vi "Main.vi"() -> ()   [LabVIEW 2020]
uses:
  <vilib>/High Genius/HG_WSI_Tookit/Dependencies/Library/CAN/CAN.lvclass
  C:/Program Files (x86)/National Instruments/LabVIEW 2020/vi.lib/High Genius/HG_WSI_Tookit/Dependencies/Library/HG_LIB/HG_LIB.lvclass
  <vilib>/High Genius/HG_WSI_Tookit/Dependencies/Library/PWM/PWM.lvclass
  <vilib>/High Genius/HG_WSI_Tookit/Dependencies/Library/Analog In/Analog In.lvclass
  <vilib>/High Genius/HG_WSI_Tookit/Dependencies/Library/Pulse/Pulse.lvclass
  <vilib>/High Genius/HG_WSI_Tookit/Dependencies/Library/ISQ/ISQ.lvclass
  <vilib>/High Genius/HG_WSI_Tookit/Dependencies/Library/IIC/IIC.lvclass
  <vilib>/High Genius/HG_WSI_Tookit/Dependencies/Library/IMU/IMU.lvclass
  <vilib>/High Genius/HG_WSI_Tookit/Dependencies/Library/Digital Input and Output/Digital Input and Output.lvclass
  <vilib>/Platform/TimedLoop/XDataNode/timing_clust.ctl
  <vilib>/Platform/TimedLoop/XDataNode/nitl_modes.ctl
  <vilib>/Platform/TimedLoop/XDataNode/wakeup.ctl
  <vilib>/Platform/TimedLoop/XDataNode/XDataNode.xnode
  <vilib>/High Genius/HG_WSI_Tookit/Dependencies/Library/HG_LIB/HG_LIB.lvclass
  <vilib>/Platform/TimedLoop/XDataNode/XDNodeRunTimeDep.lvlib
panel:
  in  "Reset Yaw":bool
  out "NavX Yaw (Rad)":dbl
  out "Ultrasonic Distance":dbl
  out "Sharp IR Distance":dbl
  out "Sharp IR Voltage":dbl
  in  "Stop Button":bool
  in  "In A":bool
  in  "In B":bool
  in  "Motor Duty Cycle":dbl(slide) scale=0.0..255.0
  out "NavX Data":dbl[](array[numeric])
  out "Cobra Values":dbl[](array[numeric])
  out "Push Button":bool
  out "Loop Number":i32
  in  "Ultrasonic Pulse":i32=20 min=0 step=1
  in  "Servo PWM":dbl(slide) min=-150.0 max=255.0 step=1.0 scale=-150.0..150.0
  # "S1"
  # "S2"
  # "S3"
  # "S4"
  # "Yaw"
  # "Pitch"
  # "Roll"
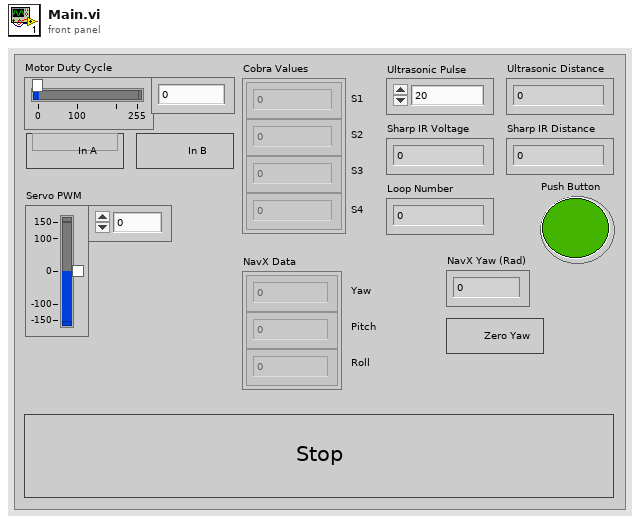
[diagram p1: front panel]
types:
  T1 = enum16{"0", "1", "2", "3", "4", "5", "6", "7", "8", "9", "10", "11", "12", "13", "14", "15", "16", "17", "18", "19", "20", "21", "22", "23", "24", "25"}
  T2 = enum16{"DI", "DO", "AI", "Pulse", "PWM", "ISQ", "ENC", "CAN", "IIC", "IMU"}
  T3 = typedef "XDNodeRunTimeDep.lvlib/timing_clust.ctl" = cluster{"Expected End [f-1]":u64, "Actual End [f-1]":u64, "Finished Late? [f-1]":bool, "Expected End [i-1]":u64, "Actual End [i-1]":u64, "Finished Late? [i-1]":bool, "Expected Start [i]":u64, "Actual Start [i]":u64, "Expected Start [f]":u64, "Actual Start [f]":u64, "Source Name":string, "Structure Name":string, "Period":i64, "Deadline":i64, "Offset":i64, "Start":i64, "Priority":i32, "Timeout":i32, "Mode":T4, "Wakeup Reason":T5, "Error":errorcluster, "Source Type":string, "Secondary Source Type":string, "Global End Time":u64, "Global Start Time":u64, "Frame Duration":u64, "Iteration Duration":u64, "Assigned CPU":i32, "I/O Scan Engine Mode":u32}
  T4 = typedef "XDNodeRunTimeDep.lvlib/nitl_modes.ctl" = enum32{"No Change", "Process missed periods, maintain original phase", "Discard missed periods, maintain original phase", "Process missed periods, ignore original phase", "Discard missed periods, ignore original phase"}
  T5 = typedef "XDNodeRunTimeDep.lvlib/wakeup.ctl" = enum32{"Normal", "Aborted", "Asynchronous wakeup", "Timing source error", "Timed loop error", "Timeout"}
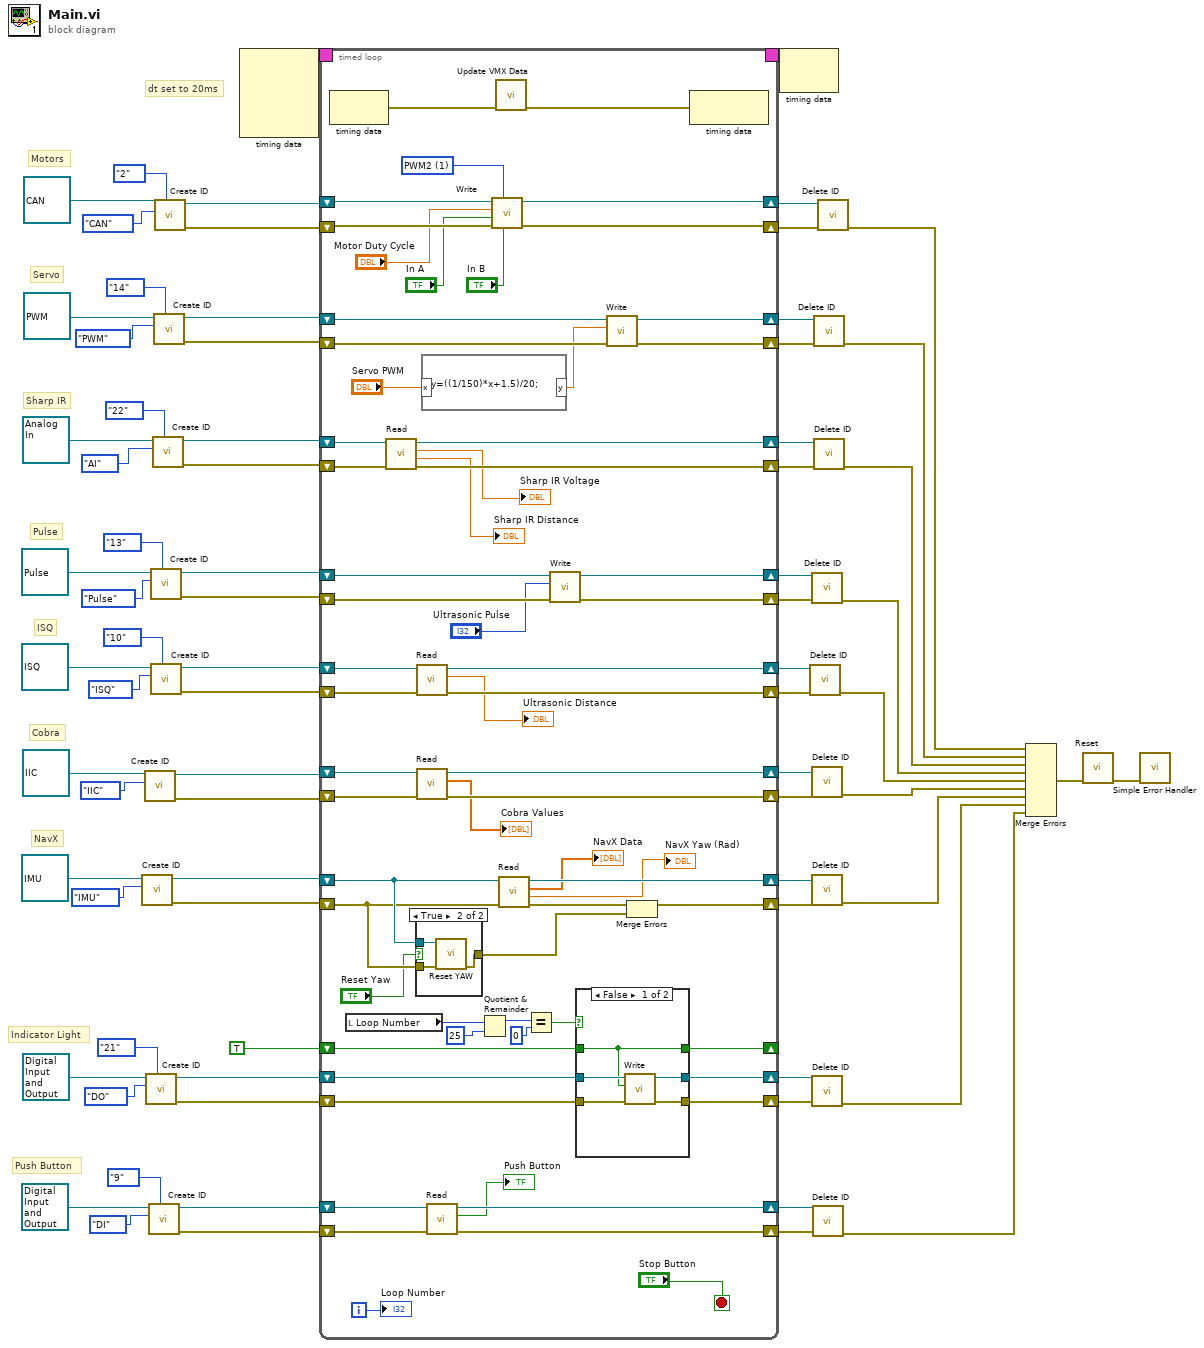
[diagram p0: block diagram]
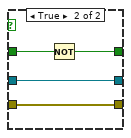
[diagram p2: hidden frame]
diagram:
  # "Push Button"
  # "Indicator Light"
  # "NavX"
  # "Cobra"
  # "ISQ"
  # "Pulse"
  # "Sharp IR"
  # "Servo"
  # "Motors"
  # "dt set to 20ms"
  n1 = call <vilib>:"Create ID.vi"("Function"=T2."IMU", "HG_LIB in"=refnum<class "IMU.lvclass"> refnum ("VMX Library.lvlib:IMU.lvclass")) -> ("error out"=w19:errorcluster, "HG_LIB out"=w20:refnum<class "IMU.lvclass">)  [unwired: 8 in]
  n2 = call <vilib>:"Create ID.vi"("Function"=T2."IIC", "HG_LIB in"=refnum<class "IIC.lvclass"> refnum ("VMX Library.lvlib:IIC.lvclass")) -> ("error out"=w26:errorcluster, "HG_LIB out"=w27:refnum<class "IIC.lvclass">)  [unwired: 8 in]
  n3 = call <vilib>:"Create ID.vi"("NO"=T1."21", "Function"=T2."DO", "HG_LIB in"=refnum<class "Digital Input and Output.lvclass"> refnum ("VMX Library.lvlib:Digital Input and Output.lvclass")) -> ("error out"=w10:errorcluster, "HG_LIB out"=w11:refnum<class "Digital Input and Output.lvclass">)  [unwired: 7 in]
  n4 = call <vilib>:"Create ID.vi"("NO"=T1."9", "Function"=T2."DI", "HG_LIB in"=refnum<class "Digital Input and Output.lvclass"> refnum ("VMX Library.lvlib:Digital Input and Output.lvclass")) -> ("error out"=w2:errorcluster, "HG_LIB out"=w3:refnum<class "Digital Input and Output.lvclass">)  [unwired: 7 in]
  n5 = call <vilib>:"Create ID.vi"("NO"=T1."13", "Function"=T2."Pulse", "HG_LIB in"=refnum<class "Pulse.lvclass"> refnum ("VMX Library.lvlib:Pulse.lvclass")) -> ("error out"=w42:errorcluster, "HG_LIB out"=w43:refnum<class "Pulse.lvclass">)  [unwired: 7 in]
  n6 = call <vilib>:"Create ID.vi"("NO"=T1."10", "Function"=T2."ISQ", "HG_LIB in"=refnum<class "ISQ.lvclass"> refnum ("VMX Library.lvlib:ISQ.lvclass")) -> ("error out"=w36:errorcluster, "HG_LIB out"=w37:refnum<class "ISQ.lvclass">)  [unwired: 7 in]
  n7 = call <vilib>:"Create ID.vi"("NO"=T1."22", "Function"=T2."AI", "HG_LIB in"=refnum<class "Analog In.lvclass"> refnum ("VMX Library.lvlib:Analog In.lvclass")) -> ("error out"=w49:errorcluster, "HG_LIB out"=w51:refnum<class "Analog In.lvclass">)  [unwired: 7 in]
  n8 = call <vilib>:"Create ID.vi"("NO"=T1."14", "Function"=T2."PWM", "HG_LIB in"=refnum<class "PWM.lvclass"> refnum ("VMX Library.lvlib:PWM.lvclass")) -> ("error out"=w60:errorcluster, "HG_LIB out"=w59:refnum<class "PWM.lvclass">)  [unwired: 7 in]
  n9 = call <vilib>:"Create ID.vi"("NO"=T1."2", "Function"=T2."CAN", "HG_LIB in"=refnum<class "CAN.lvclass"> refnum ("VMX Library.lvlib:CAN.lvclass")) -> ("error out"=w69:errorcluster, "HG_LIB out"=w68:refnum<class "CAN.lvclass">)  [unwired: 7 in]
  n10 = node-c288() -> (w75:T3)  [unwired: 4 in]
  n11 = timed-loop {
    timing: w75 -> [_]
    timing-out: [_] -> w74
    shift-right: [w136] -> w71
    shift-left: w69 -> [w134]
    shift-right: [w137] -> w72
    shift-left: w68 -> [w135]
    shift-right: [w132] -> w62
    shift-left: w60 -> [w129]
    shift-right: [w131] -> w61
    shift-left: w59 -> [w130]
    shift-right: [w128] -> w52
    shift-left: w51 -> [w127]
    shift-right: [w126] -> w50
    shift-left: w49 -> [w125]
    shift-right: [w124] -> w45
    shift-left: w43 -> [w122]
    shift-right: [w123] -> w44
    shift-left: w42 -> [w121]
    shift-right: [w119] -> w39
    shift-left: w37 -> [w117]
    shift-right: [w118] -> w38
    shift-left: w36 -> [w116]
    shift-right: [w115] -> w29
    shift-left: w27 -> [w113]
    shift-right: [w114] -> w28
    shift-left: w26 -> [w112]
    shift-right: [w111] -> w24
    shift-left: w20 -> [w110]
    shift-right: [w106] -> w23
    shift-left: w19 -> [w109]
    shift-right: [w99] -> _
    shift-left: TRUE -> [w100]
    shift-right: [w98] -> w13
    shift-left: w11 -> [w96]
    shift-right: [w97] -> w12
    shift-left: w10 -> [w95]
    shift-right: [w94] -> w5
    shift-left: w3 -> [w92]
    shift-right: [w93] -> w4
    shift-left: w2 -> [w91]
    i -> [w90]
    stop <- "Stop Button" stop-if-true
    w133 = u16 1 items=["PWM1", "PWM2", "PWM3", "PWM4"] ("PWM")
    n12 = node-c288() -> (w138:errorcluster)  [unwired: 1 in]
    n13 = local read "Loop Number"() -> (w105:i32)
    n14 = call <vilib>:"Read.vi"("error in (no error)"=w125, "Analog In in"=w127) -> ("error out"=w126:errorcluster, "IR"=→"Sharp IR Distance":dbl, "Data"=→"Sharp IR Voltage":dbl, "Analog In out"=w128:refnum<class "Analog In.lvclass">)  [unwired: 6 in]
    n15 = case shown="True" "Reset Yaw" {
      tunnel: w110 -> [_ w152]
      tunnel: w109 -> [w149 w151]
      tunnel: [w149 w150] -> w108
      frame False {
      }
      frame True {
        n16 = call <vilib>:"Reset YAW.vi"("error in (no error)"=w151, "IMU in"=w152) -> ("error out"=w150:errorcluster)  [unwired: 8 in, 1 out]
      }
    }
    n17 = call <vilib>:"Read.vi"("error in (no error)"=w116, "ISQ in"=w117) -> ("error out"=w118:errorcluster, "PING"=→"Ultrasonic Distance":dbl, "ISQ out"=w119:refnum<class "ISQ.lvclass">)  [unwired: 7 in]
    n18 = call <vilib>:"Read.vi"("error in (no error)"=w112, "IIC in"=w113) -> ("error out"=w114:errorcluster, "QTI"=→"Cobra Values":dbl[], "IIC out"=w115:refnum<class "IIC.lvclass">)  [unwired: 7 in]
    n19 = formula code="y=((1/150)*x+1.5)/20;"("x"="Servo PWM") -> ("y"=w76:dbl)
    n20 = call <vilib>:"Read.vi"("error in (no error)"=w91, "Digital Input and Output in"=w92) -> ("error out"=w93:errorcluster, "Boolean"=→"Push Button":bool, "Digital Input and Output out"=w94:refnum<class "Digital Input and Output.lvclass">)  [unwired: 7 in]
    n21 = Quotient & Remainder(x=w105, y=25) -> (x-y*floor(x/y)=w103:i32)  [unwired: 1 out]
    n22 = call <vilib>:"Write.vi"("INB"="In B", "PWM"=w133, "error in (no error)"=w134, "INA"="In A", "Duty Cycle"="Motor Duty Cycle", "CAN in"=w135) -> ("error out"=w136:errorcluster, "CAN out"=w137:refnum<class "CAN.lvclass">)  [unwired: 4 in]
    n23 = call <vilib>:"Update VMX Data.vi"("error in (no error)"=w138) -> ("error out"=w139:errorcluster)  [unwired: 10 in]
    n24 = call <vilib>:"Read.vi"("error in (no error)"=w109, "IMU in"=w110) -> ("error out"=w107:errorcluster, "YAW (rad)"=→"NavX Yaw (Rad)":dbl, "IMU"=→"NavX Data":dbl[], "IMU out"=w111:refnum<class "IMU.lvclass">)  [unwired: 6 in]
    n25 = Equal?(x=w103, y=0) -> (x = y?=w101:bool)
    n26 = call <vilib>:"Write.vi"("error in (no error)"=w121, "Pulse"="Ultrasonic Pulse", "Pulse in"=w122) -> ("error out"=w123:errorcluster, "Pulse out"=w124:refnum<class "Pulse.lvclass">)  [unwired: 7 in]
    n27 = case shown="False" w101 {
      tunnel: w100 -> [w140 w148]
      tunnel: [w140 w147] -> w99
      tunnel: [w144 w146] -> w98
      tunnel: [w143 w145] -> w97
      tunnel: w96 -> [w142 w146]
      tunnel: w95 -> [w141 w145]
      frame False {
        n28 = call <vilib>:"Write.vi"("error in (no error)"=w141, "Control"=w140, "Digital Input and Output in"=w142) -> ("error out"=w143:errorcluster, "Digital Input and Output out"=w144:refnum<class "Digital Input and Output.lvclass">)  [unwired: 7 in]
      }
      frame True {
        n29 = Not(x=w148) -> (.not. x?=w147:bool)
      }
    }
    n30 = call <vilib>:"Write.vi"("error in (no error)"=w129, "PWM"=w76, "PWM in"=w130) -> ("error out"=w132:errorcluster, "PWM out"=w131:refnum<class "PWM.lvclass">)  [unwired: 7 in]
    n31 = Merge Errors(w107, w108) -> (w106:errorcluster)
    n32 = node-c288(w139) -> ()  [unwired: 1 out]
    "Loop Number" <- w90
  }
  n33 = node-c288(w74) -> ()  [unwired: 1 out]
  n34 = call <vilib>:"Delete ID.vi"("error in (no error)"=w38, "HG_LIB in"=w39) -> ("error out"=w32:errorcluster)  [unwired: 8 in, 1 out]
  n35 = call <vilib>:"Delete ID.vi"("error in (no error)"=w44, "HG_LIB in"=w45) -> ("error out"=w33:errorcluster)  [unwired: 8 in, 1 out]
  n36 = call <vilib>:"Delete ID.vi"("error in (no error)"=w28, "HG_LIB in"=w29) -> ("error out"=w25:errorcluster)  [unwired: 8 in, 1 out]
  n37 = call <vilib>:"Delete ID.vi"("error in (no error)"=w23, "HG_LIB in"=w24) -> ("error out"=w18:errorcluster)  [unwired: 8 in, 1 out]
  n38 = call <vilib>:"Delete ID.vi"("error in (no error)"=w12, "HG_LIB in"=w13) -> ("error out"=w9:errorcluster)  [unwired: 8 in, 1 out]
  n39 = call <vilib>:"Delete ID.vi"("error in (no error)"=w4, "HG_LIB in"=w5) -> ("error out"=w1:errorcluster)  [unwired: 8 in, 1 out]
  n40 = call <vilib>:"Delete ID.vi"("error in (no error)"=w62, "HG_LIB in"=w61) -> ("error out"=w63:errorcluster)  [unwired: 8 in, 1 out]
  n41 = call <vilib>:"Delete ID.vi"("error in (no error)"=w50, "HG_LIB in"=w52) -> ("error out"=w48:errorcluster)  [unwired: 8 in, 1 out]
  n42 = call <vilib>:"Delete ID.vi"("error in (no error)"=w71, "HG_LIB in"=w72) -> ("error out"=w64:errorcluster)  [unwired: 8 in, 1 out]
  n43 = Merge Errors(w64, w63, w48, w33, w32, w25, w18, w9, w1) -> (w65:errorcluster)
  n44 = call <vilib>:"Reset.vi"("error in (no error)"=w65) -> ("error out"=w73:errorcluster)  [unwired: 10 in]
  n45 = call <vilib>:"Simple Error Handler.vi"("error in (no error)"=w73) -> ()  [unwired: 4 in, 5 out]
